vi "Send Steps.vi"(8 "error in (no error)":errorcluster, 9 "Write Data?":bool=TRUE, 10 "Command.Steps":i32, 11 "Model in":refnum<class "Model.lvclass">) -> (0 "error out":errorcluster, 2 "Is Force Outside of Range?":bool, 3 "Model out":refnum<class "Model.lvclass">)   [LabVIEW 2016, in "Model.lvclass"]
uses:
  Model.lvclass
  <vilib>/Platform/TimedLoop/XDataNode/timing_clust.ctl
  <vilib>/Platform/TimedLoop/XDataNode/nitl_modes.ctl
  <vilib>/Platform/TimedLoop/XDataNode/wakeup.ctl
  Model.lvclass/Model.ctl
  common_rt_hpilc/HPILC/HPILC.lvclass/HPILC.ctl
  <vilib>/platform/TimedLoop/XDataNode/XDataNode.xnode
  Modbus/DesktopModbus/DesktopModbus.lvclass
  common_rt_hpilc/HPILC/HPILC.lvclass
  <vilib>/Platform/TimedLoop/XDataNode/XDNodeRunTimeDep.lvlib
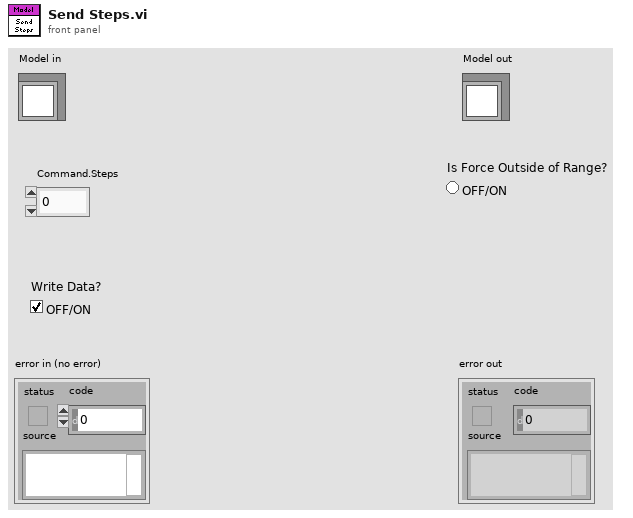
[diagram p1: front panel]
types:
  T1 = typedef "XDNodeRunTimeDep.lvlib/timing_clust.ctl" = cluster{"Expected End [f-1]":u64, "Actual End [f-1]":u64, "Finished Late? [f-1]":bool, "Expected End [i-1]":u64, "Actual End [i-1]":u64, "Finished Late? [i-1]":bool, "Expected Start [i]":u64, "Actual Start [i]":u64, "Expected Start [f]":u64, "Actual Start [f]":u64, "Source Name":string, "Structure Name":string, "Period":i64, "Deadline":i64, "Offset":i64, "Start":i64, "Priority":i32, "Timeout":i32, "Mode":T2, "Wakeup Reason":T3, "Error":errorcluster, "Source Type":string, "Secondary Source Type":string, "Global End Time":u64, "Global Start Time":u64, "Frame Duration":u64, "Iteration Duration":u64, "Assigned CPU":i32, "I/O Scan Engine Mode":u32}
  T2 = typedef "XDNodeRunTimeDep.lvlib/nitl_modes.ctl" = enum32{"No Change", "Process missed periods, maintain original phase", "Discard missed periods, maintain original phase", "Process missed periods, ignore original phase", "Discard missed periods, ignore original phase"}
  T3 = typedef "XDNodeRunTimeDep.lvlib/wakeup.ctl" = enum32{"Normal", "Aborted", "Asynchronous wakeup", "Timing source error", "Timed loop error", "Timeout"}
  T4 = typedef "RTHPILC.lvlib/HPData.ctl" = cluster{"Constants":T5, "Command":T6, "Telemetry":T7, "Responses":T8, "Timings":T10}
  T5 = typedef "RTHPILC.lvlib/HPConstants.ctl" = cluster{"ID":i16, "ReferencePosition":i32}
  T6 = typedef "RTHPILC.lvlib/HPCommand.ctl" = cluster{"Steps":i8}
  T7 = typedef "RTHPILC.lvlib/HPTelemetry.ctl" = cluster{"ILCFault":bool, "LimitSwitchCWOperated":bool, "LimitSwitchCCWOperated":bool, "BroadcastCounter":u8, "SSIEncoderValue":i32, "LoadCellForce":sgl}
  T8 = typedef "RTHPILC.lvlib/HPResponses.ctl" = cluster{"StepMotor":T9, "ForceAndStatus":T9}
  T9 = typedef "RTModbus.lvlib/ExceptionCodes.ctl" = u16
  T10 = typedef "RTHPILC.lvlib/HPTimings.ctl" = cluster{"BroadcastStepMotor":u32, "ForceAndStatus":u32, "FreezeSensorValues":u32, "StepMotor":u32}
  T11 = typedef "RTModbus.lvlib/TxFrame.ctl" = cluster{"Data":u8[], "WaitForTrigger":bool, "WaitForRx":u16, "TriggerIRQ":bool, "DelayMicroseconds":u16, "DelayMilliseconds":u16, "Timestamp":bool}
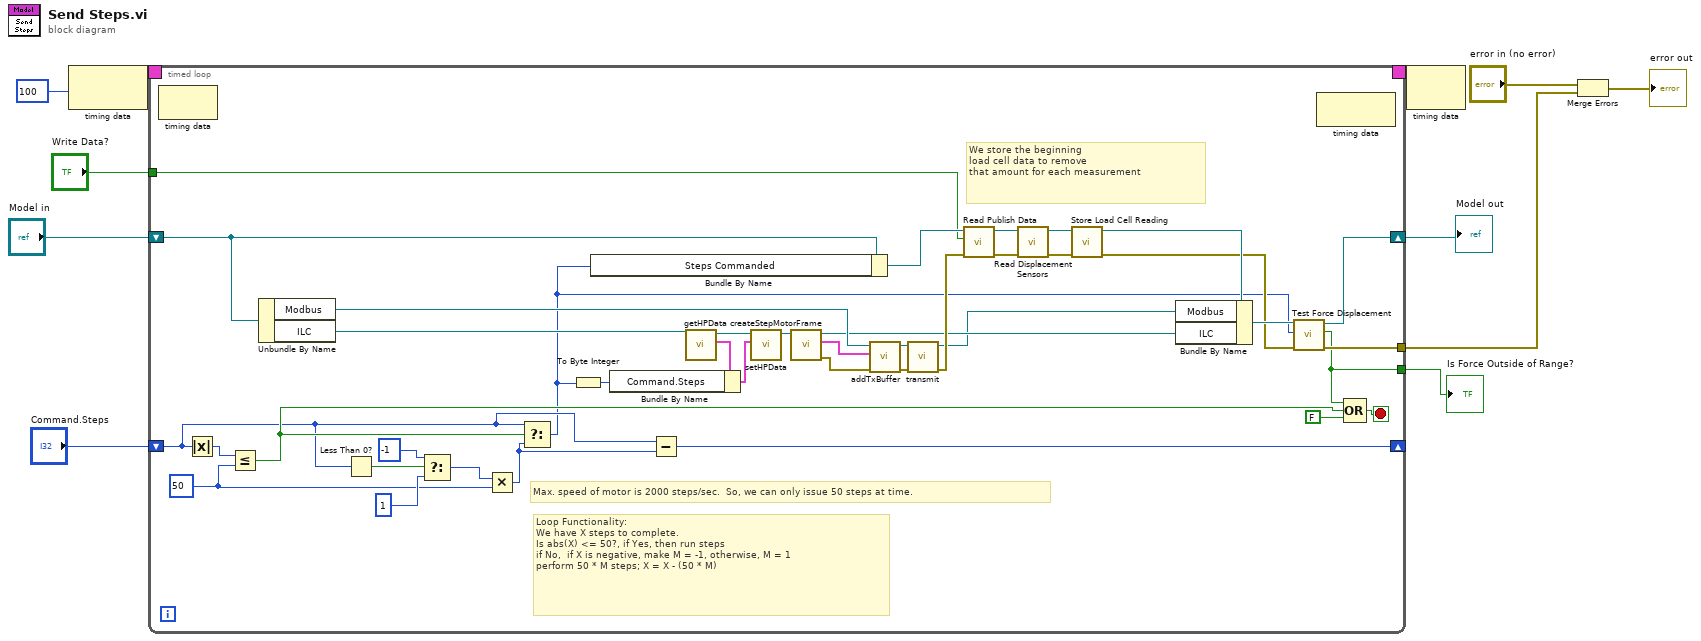
[diagram p0: block diagram]
diagram:
  n1 = node-c288(i64 100 ("Period")) -> (w7:T1)
  n2 = timed-loop {
    shift-right: [w34] -> _
    shift-left: "Command.Steps" -> [w26]
    shift-right: [w16] -> w4
    shift-left: "Model in" -> [w27]
    timing: w7 -> [_]
    timing-out: [_] -> w6
    tunnel: "Write Data?" -> [w24]
    tunnel: [w14] -> w2
    tunnel: [w13] -> w1
    stop <- w40 stop-if-true
    w37 = 50
    # "We store the beginning\nload cell data to remove\nthat amount for each measurement"
    # "Loop Functionality:\nWe have X steps to complete. \nIs abs(X) <= 50?, if Yes, then run steps\nif No,  if X is negative, make M = -1, otherwise, M = 1\nperform 50 * M steps; X = X - (50 * M)"
    # "Max. speed of motor is 2000 steps/sec.  So, we can only issue 50 steps at time."
    n3 = node-c288() -> ()  [unwired: 1 in, 1 out]
    n4 = Absolute Value(x=w26) -> (abs(x)=w43:i32)
    n5 = Less Or Equal?(x=w43, y=w37) -> (x <= y?=w33:bool)
    n6 = Unbundle By Name(w27) -> ("Modbus"=w30:refnum<class "DesktopModbus.lvclass">, "ILC"=w29:refnum<class "HPILC.lvclass">)
    n7 = Less Than 0?(x=w26) -> (x < 0?=w32:bool)
    n8 = Select(t=-1, s=w32, f=1) -> (s? t:f=w38:i32)
    n9 = Multiply(x=w38, y=w37) -> (x*y=w35:i32)
    n10 = Select(t=w26, s=w33, f=w35) -> (s? t:f=w12:i32)
    n11 = To Byte Integer(number=w12) -> (8bit integer=w36:i8)
    n12 = Bundle By Name(cluster=w27, "Steps Commanded"=w12) -> (w25:refnum<class "Model.lvclass">)
    n13 = Subtract(x=w26, y=w35) -> (x-y=w34:i32)
    n14 = call "getHPData.vi"("HPILC in"=w29) -> ("HPData"=w51:T4, "HPILC out"=w50:refnum<class "HPILC.lvclass">)  [unwired: 9 in]
    n15 = Bundle By Name(cluster=w51, "Command.Steps"=w36) -> (w44:T4)
    n16 = call "setHPData.vi"("HPData"=w44, "HPILC in"=w50) -> ("HPILC out"=w49:refnum<class "HPILC.lvclass">)  [unwired: 9 in]
    n17 = call "createStepMotorFrame.vi"("HPILC in"=w49) -> ("error out"=w46:errorcluster, "TxFrame"=w47:T11, "HPILC out"=w23:refnum<class "HPILC.lvclass">)  [unwired: 8 in]
    n18 = call-dynamic "addTxBuffer.vi"("error in (no error)"=w46, "TxFrame"=w47, "DesktopModbus in"=w30) -> ("error out"=w45:errorcluster, "DesktopModbus out"=w48:refnum<class "DesktopModbus.lvclass">)  [unwired: 7 in]
    n19 = call-dynamic "transmit.vi"("error in (no error)"=w45, "DesktopModbus in"=w48) -> ("error out"=w31:errorcluster, "DesktopModbus out"=w22:refnum<class "DesktopModbus.lvclass">)  [unwired: 8 in]
    n20 = call "Read Publish Data.vi"("error in (no error)"=w31, "Write Data?"=w24, "Model in"=w25) -> ("error out"=w19:errorcluster, "Model out"=w28:refnum<class "Model.lvclass">)  [unwired: 7 in]
    n21 = call "Read Displacement Sensors.vi"("error in (no error)"=w19, "Model in"=w28) -> ("error out"=w18:errorcluster, "Model out"=w20:refnum<class "Model.lvclass">)  [unwired: 8 in]
    n22 = call "Store Load Cell Reading.vi"("error in (no error)"=w18, "Model in"=w20) -> ("error out"=w15:errorcluster, "Model out"=w21:refnum<class "Model.lvclass">)  [unwired: 8 in]
    n23 = Bundle By Name(cluster=w21, "Modbus"=w22, "ILC"=w23) -> (w17:refnum<class "Model.lvclass">)
    n24 = call "Test Force Displacement.vi"("error in (no error)"=w15, "Number of Steps Commanded"=w12, "Model in"=w17) -> ("error out"=w14:errorcluster, "Is Force Outside of Range?"=w13:bool, "Model out"=w16:refnum<class "Model.lvclass">)  [unwired: 6 in]
    n25 = node-c288() -> ()  [unwired: 1 in, 1 out]
    n26 = Compound Arithmetic op=OR(w13, w33, FALSE) -> (w40:bool)
  }
  "Model out" <- w4
  "Is Force Outside of Range?" <- w1
  n27 = node-c288(w6) -> ()  [unwired: 1 out]
  n28 = Merge Errors("error in (no error)", w2) -> (→"error out":errorcluster)
